vi "Load Plugin.vi"(6 "Version String":string, 8 "error in (no error)":errorcluster, 9 "Unique Name":string, 10 "Plugin Type":string="CIFTemplatePlugin", 11 "Launcher in":refnum<class "CIFPluginManager.lvclass">) -> (0 "error out":errorcluster, 3 "Launcher out":refnum<class "CIFPluginManager.lvclass">)   [LabVIEW 2021, in "CIFPluginManager.lvclass"]
uses:
  CIFPluginManager.lvclass
  CIFPluginManager.lvclass/CIFPluginManager.ctl
  <vilib>/Utility/LVLibp/NI_PackedLibraryUtility.lvlib
  CIFCore/Common/Typedef/Version.ctl
  CIFCore/Common/CIFCoreCommon.lvlib
  typedef/Plugin Management Data.ctl
  CIFCore/Common/Typedef/Errors.ctl
  <vilib>/gRPC/LabVIEW gRPC Library/Shared/grpcId.ctl
  <vilib>/gRPC/LabVIEW gRPC Library/grpc-lvsupport-release.lvlib
  gRPC/CIF_Manager_server/RPC Messages/cif_plugincore_MonitorI64.ctl
  gRPC/CIF_Manager_server/CIF_Manager_server.lvlib
  gRPC/CIF_Manager_server/RPC Messages/cif_plugincore_MonitorU64.ctl
  gRPC/CIF_Manager_server/RPC Messages/cif_plugincore_MonitorDoubles.ctl
  gRPC/CIF_Manager_server/RPC Messages/cif_plugincore_Error.ctl
  gRPC/CIF_Manager_server/RPC Messages/cif_plugincore_TimingStatsBasic.ctl
  gRPC/CIF_Manager_server/RPC Messages/cif_plugincore_FifoStatistics.ctl
  gRPC/CIF_Manager_server/RPC Messages/cif_plugincore_TimingStatistics.ctl
  gRPC/CIF_Manager_server/RPC Messages/cif_plugincore_StatusData_State.ctl
  gRPC/CIF_Manager_server/RPC Messages/cif_plugincore_StatusData.ctl
  <vilib>/CIF Foundation/CIF Utilities/Time/Time_CIF_U.lvlib
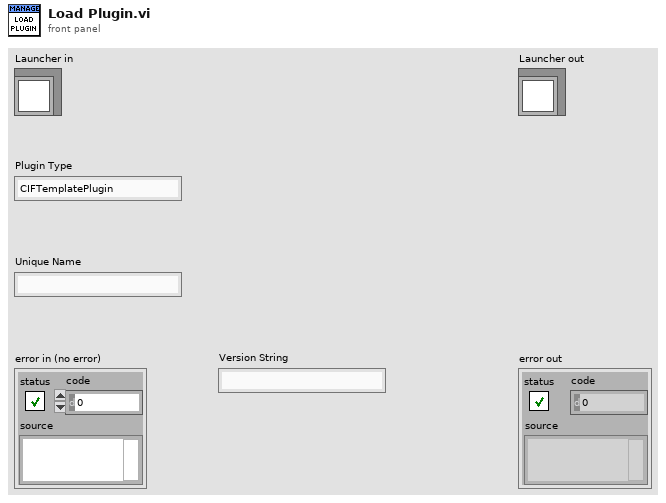
[diagram p1: front panel]
types:
  T1 = typedef "CIFCoreCommon.lvlib/Errors.ctl" = enum16{"Invalid Clock ID", "Long Sleep", "gRPC Server Not Found", "Config Parse", "Timestamp Wrap", "Delayed Execution", "Duplicate Channel", "Missing Channel", "Incorrect Type", "Flatten Error", "Unflatten Data", "Unique Name", "Plugin Not Found", "Plugin Type Not Found", "Plugin Version Not Found", "Manager Not Found", "Numerical Issue", "Time Jump", "Clock ID Match", "Channel Length", "Plugin Connection", "gRPC Server Connection", "PPL Name Match", "Build", "Config Log Parse"}
  T2 = typedef "CIFPluginManager.lvclass/Plugin Management Data.ctl" = cluster{"vi reference":refnum<vi>, "gRPC ID":T3, "Plugin Type":string, "Unique Name":string, "gRPC Port":i32, "Version":T4, "Load Timestamp":i64, "Unload Timestamp":i64, "Unloading":bool, "Ready for removal":bool, "status":T5}
  T3 = typedef "grpc-lvsupport-release.lvlib/grpcId.ctl" = u64
  T4 = typedef "CIFCoreCommon.lvlib/Version.ctl" = cluster{"Major":i32, "Minor":i32, "Fix":i32, "Build":i32}
  T5 = typedef "CIF_Manager_server.lvlib/cif_plugincore_StatusData.ctl" = cluster{"state":T6, "timing_statistics":T7, "fifo_statistics":T9, "error":T10, "monitor_doubles":T11, "monitor_u64s":T12, "monitor_i64s":T13}
  T6 = typedef "CIF_Manager_server.lvlib/cif_plugincore_StatusData_State.ctl" = enum32{"NULL", "CREATING", "LISTENING", "RUNNING", "CLEANINGUP", "DESTROYING"}
  T7 = typedef "CIF_Manager_server.lvlib/cif_plugincore_TimingStatistics.ctl" = cluster{"period":T8, "wake_error":T8, "execute":T8, "housekeep":T8, "idle":T8, "cleanup":T8, "custom_1":T8, "custom_2":T8}
  T8 = typedef "CIF_Manager_server.lvlib/cif_plugincore_TimingStatsBasic.ctl" = cluster{"max":i64, "min":i64, "avg":dbl}
  T9 = typedef "CIF_Manager_server.lvlib/cif_plugincore_FifoStatistics.ctl" = cluster{"from_t0":T8, "from_previous_plugin":T8, "output_error":T8}
  T10 = typedef "CIF_Manager_server.lvlib/cif_plugincore_Error.ctl" = cluster{"status":bool, "code":i32}
  T11 = typedef "CIF_Manager_server.lvlib/cif_plugincore_MonitorDoubles.ctl" = cluster{"double_1":dbl, "double_2":dbl, "double_3":dbl, "double_4":dbl}
  T12 = typedef "CIF_Manager_server.lvlib/cif_plugincore_MonitorU64.ctl" = cluster{"u64_1":u64, "u64_2":u64, "u64_3":u64, "u64_4":u64}
  T13 = typedef "CIF_Manager_server.lvlib/cif_plugincore_MonitorI64.ctl" = cluster{"i64_1":i64, "i64_2":i64, "i64_3":i64, "i64_4":i64}
  T14 = typedef "CIFPluginManager.lvclass/Discovered Plugin.ctl" = cluster{"Filename":string, "Plugin Type":string, "Qualified name":string, "Version":T4}
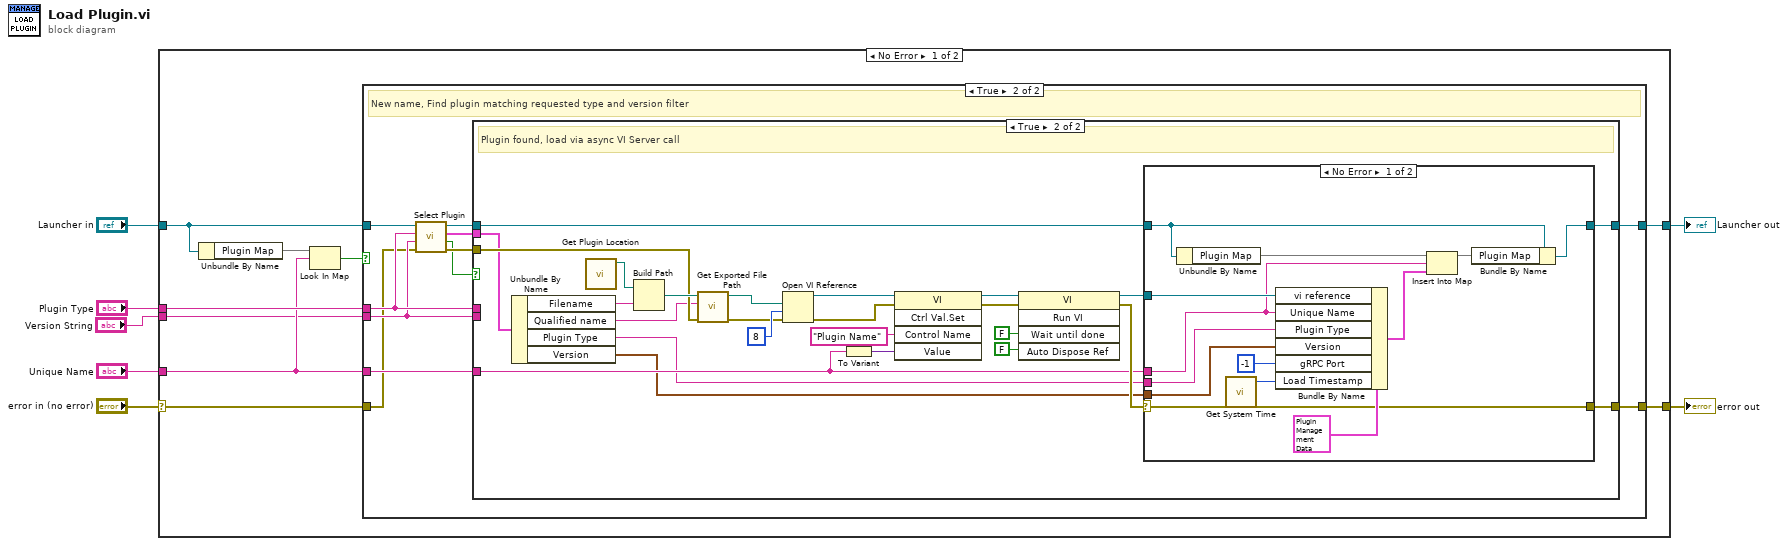
[diagram p0: block diagram]
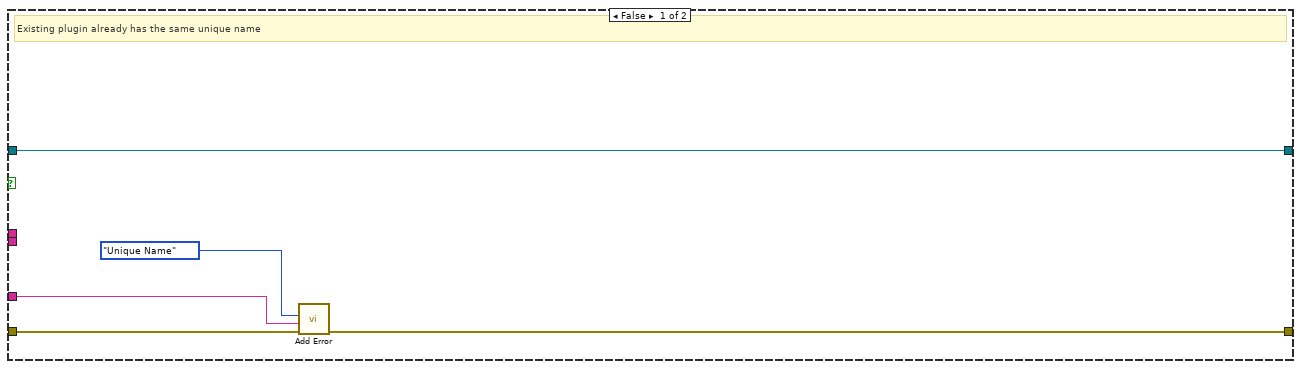
[diagram p2: hidden frame]
diagram:
  n1 = case shown="No Error" "error in (no error)" {
    selector: "error in (no error)" -> [w16 w76]
    tunnel: [w15 w76] -> w6
    tunnel: [w11 w75] -> w4
    tunnel: "Launcher in" -> [w8 w75]
    tunnel: "Plugin Type" -> [w14 _]
    tunnel: "Unique Name" -> [w13 _]
    tunnel: "Version String" -> [w9 _]
    frame No Error {
      n2 = Unbundle By Name(w8) -> ("Plugin Map"=w12:map{string, T2})
      n3 = Look In Map(map=w12, key=w13) -> (key not found?=w10:bool)  [unwired: 1 in, 1 out]
      n4 = case shown="True" w10 {
        tunnel: w16 -> [w21 w25]
        tunnel: [w18 w31] -> w15
        tunnel: w14 -> [_ w27]
        tunnel: w13 -> [w19 w32]
        tunnel: w8 -> [w17 w29]
        tunnel: [w17 w30] -> w11
        tunnel: w9 -> [_ w26]
        frame False {
          # "Existing plugin already has the same unique name"
          n5 = call "Add Error.vi"("error in (no error)"=w21, "String to Append"=w19, "Error"=Errors."Unique Name") -> ("error out"=w18:errorcluster)  [unwired: 8 in]
        }
        frame True {
          # "New name, Find plugin matching requested type and version filter"
          n6 = call "Select Plugin.vi"("error in (no error)"=w25, "Version String"=w26, "Plugin Type"=w27, "CIFPluginManager in"=w29) -> ("error out"=w24:errorcluster, "Match found"=w23:bool, "Matching Plugin"=w22:T14, "CIFPluginManager out"=w28:refnum<class "CIFPluginManager.lvclass">)  [unwired: 4 in]
          n7 = case shown="True" w23 {
            tunnel: w32 -> [_ w45]
            tunnel: [w33 w44] -> w31
            tunnel: [w34 w43] -> w30
            tunnel: w28 -> [w34 w41]
            tunnel: w27 -> [_ _]
            tunnel: w26 -> [_ _]
            tunnel: w24 -> [w33 w40]
            tunnel: w22 -> [_ w39]
            frame False {
              # "Plugin not found"
            }
            frame True {
              # "Plugin found, load via async VI Server call"
              n8 = Unbundle By Name(w39) -> ("Filename"=w38:string, "Qualified name"=w37:string, "Plugin Type"=w36:string, "Version"=w35:T4)
              n9 = call "Get Plugin Location.vi"() -> ("Plugin Directory"=w42:path)  [unwired: 11 in]
              n10 = Build Path(base path=w42, name or relative path=w38) -> (appended path=w59:path)
              n11 = call <vilib>:"Get Exported File Path.vi"("error in (no error)"=w40, "qualified name"=w37, "packed library path"=w59) -> ("error out"=w50:errorcluster, "path"=w51:path)  [unwired: 7 in]
              n12 = Open VI Reference(vi path=w51, options=8, error in (no error)=w50) -> (vi reference=w53:refnum<vi>, error out=w56:errorcluster)  [unwired: 3 in]
              n13 = To Variant(anything=w45) -> (Variant=w49:variant)
              n14 = invoke class="VI" method="Ctrl Val.Set"(reference=w53, error in=w56, "Control Name"="Plugin Name", "Value"=w49) -> (reference out=w55:refnum<vi>, error out=w54:errorcluster)  [unwired: 1 in, 3 out]
              n15 = invoke class="VI" method="Run VI"(reference=w55, error in=w54, "Wait until done"=FALSE ("Wait Until Done"), "Auto Dispose Ref"=FALSE ("Auto Dispose Reference")) -> (reference out=w46:refnum<vi>, error out=w47:errorcluster)  [unwired: 1 in, 3 out]
              n16 = case shown="No Error" w47 {
                selector: w47 -> [w61 w73]
                tunnel: w46 -> [w72 _]
                tunnel: w45 -> [w68 _]
                tunnel: w41 -> [w66 w74]
                tunnel: [w61 w73] -> w44
                tunnel: w36 -> [w70 _]
                tunnel: [w64 w74] -> w43
                tunnel: w35 -> [w63 _]
                frame No Error {
                  n17 = Unbundle By Name(w66) -> ("Plugin Map"=w69:map{string, T2})
                  n18 = call <vilib>:"Get System Time.vi"() -> ("Time (ns)"=w60:i64)  [unwired: 5 in]
                  n19 = Bundle By Name(cluster=T2 {"vi reference"=refnum, "gRPC ID"=0, "Plugin Type"="", "Unique Name"="", "gRPC Port"=0, "Version"={"Major"=0, "Minor"=0, "Fix"=0, "Build"=0}, "Load Timestamp"=0, "Unload Timestamp"=0, "Unloading"=FALSE, "Ready for removal"=FALSE, "status"={"state"=enum."NULL", "timing_statistics"={"period"={"max"=0, "min"=0, "avg"=0.0}, "wake_error"={"max"=0, "min"=0, "avg"=0.0}, "execute"={"max"=0, "min"=0, "avg"=0.0}, "housekeep"={"max"=0, "min"=0, "avg"=0.0}, "idle"={"max"=0, "min"=0, "avg"=0.0}, "cleanup"={"max"=0, "min"=0, "avg"=0.0}, "custom_1"={"max"=0, "min"=0, "avg"=0.0}, "custom_2"={"max"=0, "min"=0, "avg"=0.0}}, "fifo_statistics"={"from_t0"={"max"=0, "min"=0, "avg"=0.0}, "from_previous_plugin"={"max"=0, "min"=0, "avg"=0.0}, "output_error"={"max"=0, "min"=0, "avg"=0.0}}, "error"={"status"=FALSE, "code"=0}, "monitor_doubles"={"double_1"=0.0, "double_2"=0.0, "double_3"=0.0, "double_4"=0.0}, "monitor_u64s"={"u64_1"=0, "u64_2"=0, "u64_3"=0, "u64_4"=0}, "monitor_i64s"={"i64_1"=0, "i64_2"=0, "i64_3"=0, "i64_4"=0}}} ("Plugin Management Data"), "vi reference"=w72, "Unique Name"=w68, "Plugin Type"=w70, "Version"=w63, "gRPC Port"=-1, "Load Timestamp"=w60) -> (w67:T2)
                  n20 = Insert Into Map(map in=w69, key=w68, value=w67) -> (map out=w65:map{string, T2})  [unwired: 2 out]
                  n21 = Bundle By Name(cluster=w66, "Plugin Map"=w65) -> (w64:refnum<class "CIFPluginManager.lvclass">)
                }
                frame Error {
                }
              }
            }
          }
        }
      }
    }
    frame Error {
    }
  }
  "error out" <- w6
  "Launcher out" <- w4
